vi "002 Conversió unitats cluster tres elements.vi"() -> ()   [LabVIEW 2019]
panel:
  out "Cluster":T1 {"Gauge" scale=0.0..100000.0; "Tank" scale=0.0..100.0; "Thermometer" scale=0.0..500.0}
  in  "Variables sense escalar":T2
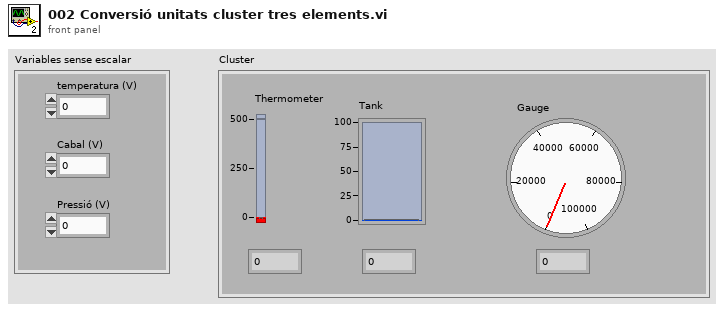
[diagram p1: front panel]
types:
  T1 = cluster{"Thermometer":dbl, "Tank":dbl, "Gauge":dbl}
  T2 = cluster{"temperatura (V)":dbl, "Cabal (V)":dbl, "Pressió (V)":dbl}
  T3 = cluster{"Cº/V":dbl, "(litres/s)/V":dbl, "(N/m^2)/V":dbl}
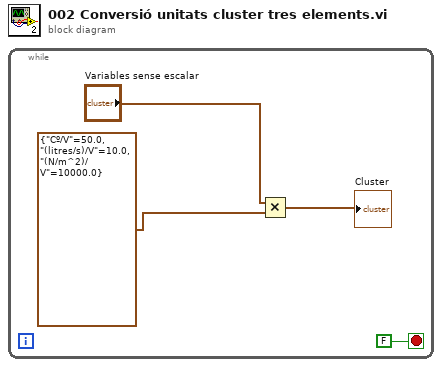
[diagram p0: block diagram]
diagram:
  n1 = while {
    stop <- FALSE stop-if-true
    n2 = Multiply(x="Variables sense escalar", y=T3 {"Cº/V"=50.0, "(litres/s)/V"=10.0, "(N/m^2)/V"=10000.0}) -> (x*y=→"Cluster":cluster{dbl, dbl, dbl})
  }
